vi "Byte Order Marks.vi"() -> (0 "BOMs":map{T1, string}(c390)={enum."UTF-8"="﻿", enum."UTF-16LE"="ÿþ", enum."UTF-16BE"="þÿ"})   [LabVIEW 2020, in "G-Unicode.lvlib"]
uses:
  G-Unicode.lvlib
  Controls/String Encoding.ctl
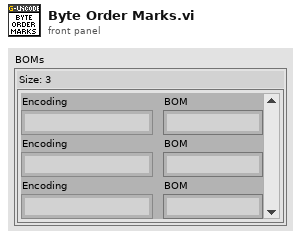
[diagram p1: front panel]
types:
  T1 = typedef "G-Unicode.lvlib/String Encoding.ctl" = enum16{"ANSI", "UTF-8", "UTF-16LE", "UTF-16BE", "Unknown"}
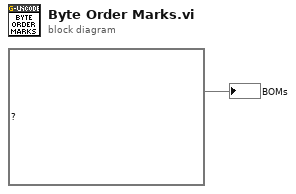
[diagram p0: block diagram]
diagram:
  "BOMs" <- map{T1, string} {enum."UTF-8"="﻿", enum."UTF-16LE"="ÿþ", enum."UTF-16BE"="þÿ"} ("map out")
